vi "CSTK_Icon_Creator_TemplateItems.vi"() -> (3 "TemplateItems":string[](array[string]))   [LabVIEW 2015, in "CSTK_Icon Creator.lvlib"]
uses:
  CSTK_Icon Creator.lvlib
  <userlib>/_OpenG.lib/array/array.llb/Search 1D Array (String)__ogtk.vi
  <userlib>/_OpenG.lib/array/array.llb/Delete Elements from 1D Array (String)__ogtk.vi
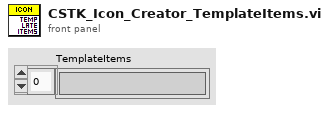
[diagram p1: front panel]
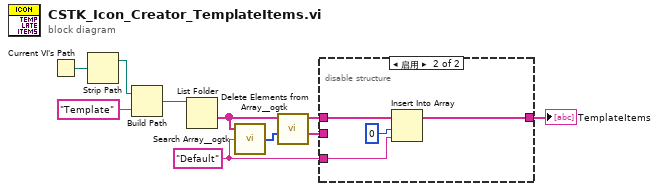
[diagram p0: block diagram]
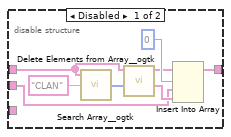
[diagram p2: hidden frame]
diagram:
  w1 = "Default" ("Element Data")
  n1 = Current VI's Path() -> (path=w2:path)
  n2 = Strip Path(path=w2) -> (stripped path=w3:path)  [unwired: 1 out]
  n3 = Build Path(base path=w3, name or relative path="Template" ("名称或相对路径")) -> (appended path=w5:path)
  n4 = List Folder(path=w5) -> (folder names=w6:string[])  [unwired: 3 in, 3 out]
  n5 = call-poly <userlib>:"Search Array__ogtk.vi"("Array"=w6, "Element Data"=w1) -> ("Indices of Elements"=w7:i32[])  [unwired: 7 in]
  n6 = call-poly <userlib>:"Delete Elements from Array__ogtk.vi"("indices"=w7, "array"=w6) -> ("deleted elements"=w9:string[], "array w/ subset deleted"=w8:string[])  [unwired: 8 in]
  n7 = disable-structure shown="启用" {
    disable-tunnel: [w17 w21] -> w10
    disable-tunnel: w9 -> [w15 _]
    disable-tunnel: w8 -> [w13 w22]
    disable-tunnel: w1 -> [_ w19]
    frame Disabled {
      n8 = call-poly <userlib>:"Search Array__ogtk.vi"("Array"=w13, "Element Data"="CLAN") -> ("Indices of Elements"=w11:i32[])  [unwired: 7 in]
      n9 = call-poly <userlib>:"Delete Elements from Array__ogtk.vi"("indices"=w11, "array"=w13) -> ("deleted elements"=w16:string[], "array w/ subset deleted"=w14:string[])  [unwired: 8 in]
      n10 = Insert Into Array(array=w14, index=0 ("索引"), new element #1=w15, new element #2=w16) -> (w17:string[])
    }
    frame Enabled {
      n11 = Insert Into Array(array=w22, index=0 ("索引"), new element=w19) -> (w21:string[])
    }
  }
  "TemplateItems" <- w10
